vi "8.8.-Momento h5.vi"(1 "n30/n12/n21/n03":dbl[](array[numeric])) -> (0 "M5":dbl)   [LabVIEW 2020]
panel:
  # "Visión Artificial - Momentos Invariantes de Hu\nDiego Cervantes Rodríguez\ndicer0.com"
  # "M5 = ((n30-3*n12)*(n30+n12)*((n30+n12)^2 -3*(n21+n03)^2))+((3*n21-n03)*(n21+n03)*(3*(n30+n12)^2 -(n21+n03)^2))"
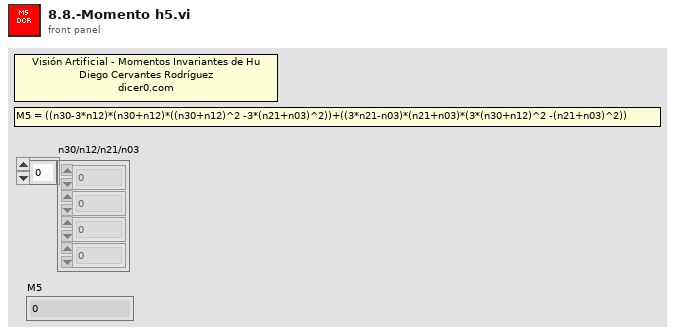
[diagram p1: front panel]
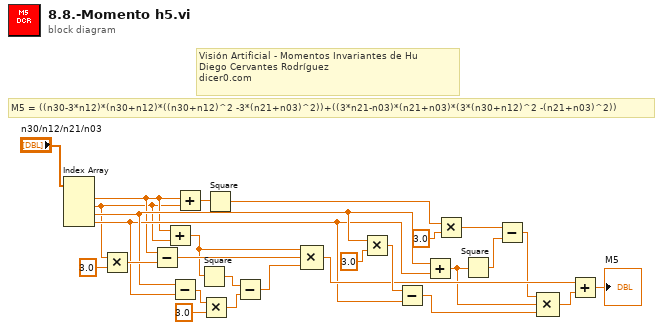
[diagram p0: block diagram]
diagram:
  # "Visión Artificial - Momentos Invariantes de Hu\nDiego Cervantes Rodríguez\ndicer0.com"
  # "M5 = ((n30-3*n12)*(n30+n12)*((n30+n12)^2 -3*(n21+n03)^2))+((3*n21-n03)*(n21+n03)*(3*(n30+n12)^2 -(n21+n03)^2))"
  n1 = Index Array "Index Array"(array="n30/n12/n21/n03") -> (element #1=w15:dbl, element #2=w14:dbl, element #3=w17:dbl, element #4=w16:dbl)  [unwired: 4 in]
  n2 = Multiply(x=w14, y=3.0) -> (x*y=w26:dbl)
  n3 = Subtract(x=w15, y=w26) -> (x-y=w21:dbl)
  n4 = Add(x=w15, y=w14) -> (x+y=w20:dbl)
  n5 = Subtract(x=w17, y=w16) -> (x-y=w25:dbl)
  n6 = Add(x=w15, y=w14) -> (x+y=w13:dbl)
  n7 = Square(x=w20) -> (x^2=w24:dbl)
  n8 = Multiply(x=w25, y=3.0) -> (x*y=w23:dbl)
  n9 = Square(x=w13) -> (x^2=w12:dbl)
  n10 = Subtract(x=w24, y=w23) -> (x-y=w22:dbl)
  n11 = Compound Arithmetic op=MULTIPLY(w20, w21, w22) -> (w18:dbl)
  n12 = Multiply(x=w17, y=3.0) -> (x*y=w19:dbl)
  n13 = Subtract(x=w19, y=w16) -> (x-y=w3:dbl)
  n14 = Add(x=w17, y=w16) -> (x+y=w2:dbl)
  n15 = Multiply(x=w12, y=3.0) -> (x*y=w10:dbl)
  n16 = Square(x=w2) -> (x^2=w9:dbl)
  n17 = Subtract(x=w10, y=w9) -> (x-y=w1:dbl)
  n18 = Compound Arithmetic op=MULTIPLY(w1, w2, w3) -> (w8:dbl)
  n19 = Add(x=w18, y=w8) -> (x+y=→"M5":dbl)
